vi "Funnel Path Points.vi"(2 "Smooth Segments":dbl, 3 "Commands":T1(array[cluster])) -> (0 "Array 2":cluster{"X":dbl, "Y":dbl}[](array[cluster]), 1 "Array":cluster{"X":dbl, "Y":dbl}[][](array[cluster]))   [LabVIEW 2016]
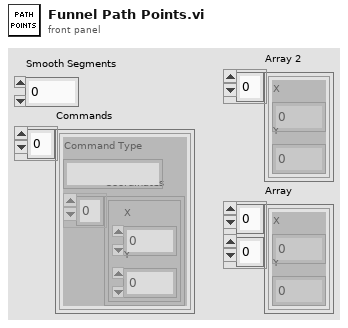
[diagram p1: front panel]
types:
  T1 = cluster{"Command Type":string, "Coordinates":cluster{"X":dbl, "Y":dbl}[]}[]
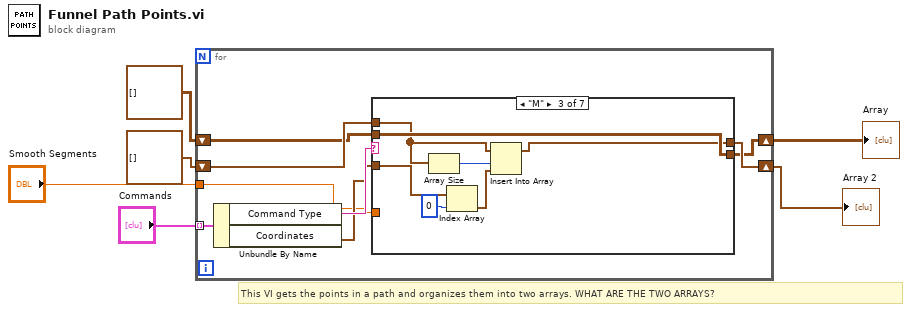
[diagram p0: block diagram]
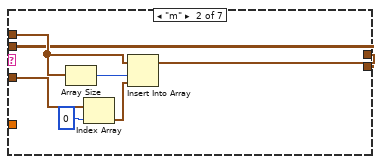
[diagram p3: hidden frame]
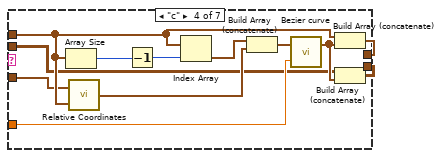
[diagram p4: hidden frame]
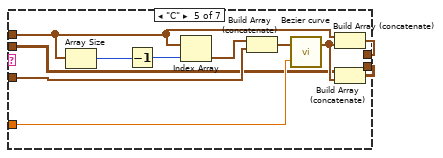
[diagram p5: hidden frame]
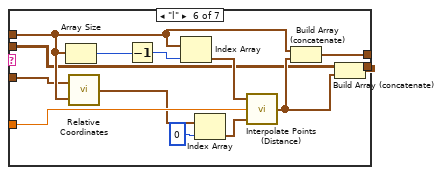
[diagram p6: hidden frame]
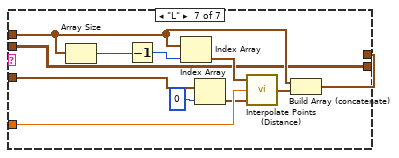
[diagram p7: hidden frame]
diagram:
  # "This VI gets the points in a path and organizes them into two arrays. WHAT ARE THE TWO ARRAYS?"
  n1 = for {
    tunnel: "Commands" -> [w14] mode=indexing
    shift-right: [w8] -> w5
    shift-left: cluster{"X":dbl, "Y":dbl}[] [] -> [w11]
    tunnel: "Smooth Segments" -> [w9]
    shift-right: [w7] -> w6
    shift-left: cluster{"X":dbl, "Y":dbl}[][] [] -> [w10]
    n2 = Unbundle By Name(w14) -> ("Command Type"=w13:string, "Coordinates"=w12:cluster{"X":dbl, "Y":dbl}[])
    n3 = case shown="\"M\"" w13 {
      tunnel: w12 -> [_ w18 w27 w34 w46 w57 w74]
      tunnel: w11 -> [w16 w20 w25 w42 w53 w59 w75]
      tunnel: [w16 w21 w24 w36 w48 w65 w76] -> w8
      tunnel: w9 -> [_ _ _ w35 w47 w66 w77]
      tunnel: [w15 w17 w26 w33 w44 w55 w67] -> w7
      tunnel: w10 -> [w15 w17 w26 w31 w43 w54 w67]
      frame "other letters", Default {
      }
      frame "m" {
        n4 = Array Size(array=w20) -> (size(s)=w23:i32)
        n5 = Index Array(array=w18, index=0) -> (element=w22:cluster{"X":dbl, "Y":dbl})
        n6 = Insert Into Array(array=w20, index=w23, new element=w22) -> (w21:cluster{"X":dbl, "Y":dbl}[])
      }
      frame "M" {
        n7 = Array Size(array=w25) -> (size(s)=w29:i32)
        n8 = Index Array(array=w27, index=0) -> (element=w28:cluster{"X":dbl, "Y":dbl})
        n9 = Insert Into Array(array=w25, index=w29, new element=w28) -> (w24:cluster{"X":dbl, "Y":dbl}[])
      }
      frame "c" {
        n10 = Array Size(array=w42) -> (size(s)=w38:i32)
        n11 = call "Relative Coordinates.vi"("All Coordinates"=w42, "Command Coordinates"=w34) -> ("Adjusted Command Coordinates"=w40:cluster{"X":dbl, "Y":dbl}[])
        n12 = Decrement(x=w38) -> (x-1=w37:i32)
        n13 = Index Array(array=w42, index=w37) -> (element=w41:cluster{"X":dbl, "Y":dbl})
        n14 = Build Array (concatenate)(w41, w40) -> (w39:cluster{"X":dbl, "Y":dbl}[])
        n15 = call "Bezier curve.vi"("Segments"=w35, "Parameters"=w39) -> ("Coordinate Array"=w32:cluster{"X":dbl, "Y":dbl}[])  [unwired: 1 out]
        n16 = Build Array (concatenate)(w42, w32) -> (w36:cluster{"X":dbl, "Y":dbl}[])
        n17 = Build Array (concatenate)(w31, w32) -> (w33:cluster{"X":dbl, "Y":dbl}[][])
      }
      frame "C" {
        n18 = Array Size(array=w53) -> (size(s)=w50:i32)
        n19 = Decrement(x=w50) -> (x-1=w49:i32)
        n20 = Index Array(array=w53, index=w49) -> (element=w52:cluster{"X":dbl, "Y":dbl})
        n21 = Build Array (concatenate)(w52, w46) -> (w51:cluster{"X":dbl, "Y":dbl}[])
        n22 = call "Bezier curve.vi"("Segments"=w47, "Parameters"=w51) -> ("Coordinate Array"=w45:cluster{"X":dbl, "Y":dbl}[])  [unwired: 1 out]
        n23 = Build Array (concatenate)(w53, w45) -> (w48:cluster{"X":dbl, "Y":dbl}[])
        n24 = Build Array (concatenate)(w43, w45) -> (w44:cluster{"X":dbl, "Y":dbl}[][])
      }
      frame "l" {
        n25 = Array Size(array=w59) -> (size(s)=w61:i32)
        n26 = call "Relative Coordinates.vi"("All Coordinates"=w59, "Command Coordinates"=w57) -> ("Adjusted Command Coordinates"=w64:cluster{"X":dbl, "Y":dbl}[])
        n27 = Decrement(x=w61) -> (x-1=w60:i32)
        n28 = Index Array(array=w59, index=w60) -> (element=w63:cluster{"X":dbl, "Y":dbl})
        n29 = Index Array(array=w64, index=0) -> (element=w62:cluster{"X":dbl, "Y":dbl})
        n30 = call "Interpolate Points (Distance).vi"("End Point"=w62, "Distance between Points"=w66, "Start Point"=w63) -> ("Output Point Array"=w56:cluster{"X":dbl, "Y":dbl}[])
        n31 = Build Array (concatenate)(w59, w56) -> (w65:cluster{"X":dbl, "Y":dbl}[])
        n32 = Build Array (concatenate)(w54, w56) -> (w55:cluster{"X":dbl, "Y":dbl}[][])
      }
      frame "L" {
        n33 = Array Size(array=w75) -> (size(s)=w70:i32)
        n34 = Decrement(x=w70) -> (x-1=w69:i32)
        n35 = Index Array(array=w75, index=w69) -> (element=w73:cluster{"X":dbl, "Y":dbl})
        n36 = Index Array(array=w74, index=0) -> (element=w71:cluster{"X":dbl, "Y":dbl})
        n37 = call "Interpolate Points (Distance).vi"("End Point"=w71, "Distance between Points"=w77, "Start Point"=w73) -> ("Output Point Array"=w68:cluster{"X":dbl, "Y":dbl}[])
        n38 = Build Array (concatenate)(w75, w68) -> (w76:cluster{"X":dbl, "Y":dbl}[])
      }
    }
  }
  "Array" <- w6
  "Array 2" <- w5
